vi "Integration Test Launcher.vi"() -> ()   [LabVIEW 2017]
doc: "<License>\nCopyright © 2017 Composed Systems, LLC | All rights reserved\nwww.composed.io\n\nAuthor: Ethan Stern <ethan.stern@composed.io>\n\nThis software is provided \"AS IS\" WITHOUT WARRANTIES, either express or implied, AND IS FOR EDUCATIONAL PURPOSES ONLY.\n</License>"
uses:
  BasicChartBinding/BasicChartBinding.lvclass
  C:/Git/mva-framework/Source/Framework/IViewable/IViewable/IViewable.lvclass
  BasicTerminalBinding/BasicTerminalBinding.lvclass
  MultiSubscriber/MultiSubscriber.lvclass
  ConcreteViewModel/ConcreteViewModel.lvclass
  C:/Git/mva-framework/Source/Framework/IObserver/IObserver/IObserver.lvclass
  C:/Git/mva-framework/Source/Framework/IViewModel/IViewModel/IViewModel.lvclass
  C:/Program Files (x86)/National Instruments/LabVIEW 2017/vi.lib/ActorFramework/Actor/Actor.lvclass
  ValueChangeEventProducer/ValueChangeEventProducer.lvclass
  BasicAutoRegistrationView/BasicAutoRegistrationView.lvclass
  ActorAutoRegistrationView/EventHandlingActor.lvclass
  Source/Framework/IViewModel/IViewModel/IViewModel.lvclass
  C:/Git/mva-framework/Source/Framework/IViewManager/IViewManager/IViewManager.lvclass
  Source/Framework/IViewable/IViewable/View Position Enum.ctl
  Source/Framework/IModel/IModel/IModel.lvclass
  Source/Framework/Mediator/Mediator/Mediator.lvclass
  C:/Git/mva-framework/Source/Framework/IMediator/IMediator/IMediator.lvclass
  <vilib>/ActorFramework/Message Enqueuer/Message Priority.ctl
  ConcreteModel/ConcreteModel.lvclass
  C:/Git/mva-framework/Source/Framework/IModel/IModel/IModel.lvclass
  Source/Framework/Mediator/MediatorBusMonitor/MediatorBusMonitor.lvclass
  C:/Git/mva-framework/Source/Framework/IMediator/IMediatorBusMonitor/IMediatorBusMonitor.lvclass
  TreeActor/TreeActor.lvclass
  MCListboxActor/MCListboxActor.lvclass
  TestApplicationStyle/TestApplicationStyle.lvclass
  <vilib>/Utility/miscctls.llb/LVPointTypeDef.ctl
  gpm_packages/@cs/event-logger/Source/Composed Log/LoggerReference/LoggerReference.lvclass/LoggerReference.ctl
  Source/Framework/IObserver/IObserver/IObserver.lvclass/IObserver.ctl
  Source/Framework/IMediator/IMediator/IMediator.lvclass/IMediator.ctl
  Source/Framework/IViewModel/IViewModel/IViewModel.lvclass/IViewModel.ctl
  Source/Framework/IViewManager/IViewManager Messages/Launch Nested Views Msg/Launch Nested Views Msg.lvclass/Launch Nested Views Msg.ctl
  Source/Framework/IViewManager/IViewManager/IViewManager.lvclass/IViewManager.ctl
  Source/Framework/IViewable/IViewable Messages/Open Front Panel Msg/Open Front Panel Msg.lvclass/Open Front Panel Msg.ctl
  <vilib>/ActorFramework/Message Enqueuer/Message Enqueuer.lvclass/Message Enqueuer.ctl
  Source/Framework/IViewable/IViewable Messages/Set Minimum Panel Size Msg/Set Minimum Panel Size Msg.lvclass/Set Minimum Panel Size Msg.ctl
  52c60252-50fc-4a03-94af-d5c5c5d06c7f.vi
  52c60252-50fc-4a03-94af-d5c5c5d06c7f.vi/977d4e1a-38bf-47f0-b12a-a53eb633355f.vi
  Source/Framework/IObserver/IObserver/Configure Observer Logging.vi
  Source/Framework/IViewModel/IViewModel/Write Startup Model-View Configuration.vi
  Source/Framework/IMediator/IMediator/Configure Mediator.vi
  <vilib>/ActorFramework/Message Enqueuer/Enqueue.vi
  gpm_packages/@cs/event-logger/Source/Composed Log/LoggerReference/Return Aggregate Queues.vi
  gpm_packages/@cs/event-logger/Source/Composed Log/LoggerReference/Add Aggregate Log.vi
  52c60252-50fc-4a03-94af-d5c5c5d06c7f.vi/977d4e1a-38bf-47f0-b12a-a53eb633355f.vi/fc2f1903-e29f-4015-abd4-fc077701cf31.vi
  Source/Framework/IViewManager/IViewManager Messages/Launch Nested Views Msg/Pack Launch Nested Views Msg.vi
  Source/Framework/IViewManager/IViewManager/Write Startup Launch Nested Views Msg.vi
  gpm_packages/@cs/event-logger/Source/Composed Log/LoggerReference/Send Add Sink.vi
  Source/ViewManager/QuadViewManager/QuadViewManager.lvclass
  Source/ViewManager/BoundViewManager/BoundViewManager.lvclass
  Source/ViewManager/TabbedViewManager/TabbedViewManager.lvclass
  Source/Framework/IViewManager/IViewManager/IViewManager.lvclass
  gpm_packages/@cs/event-logger/Source/Text File Sink/Text File Sink.lvclass
  C:/Git/mva-framework/gpm_packages/@cs/event-logger/Source/Composed Log/Log Sink/Log Sink.lvclass
  Source/ViewManager/LeftListboxViewManager/LeftListboxViewManager.lvclass
  Source/Framework/IViewable/IViewable Messages/Open Front Panel Msg/Open Front Panel Msg.lvclass
  C:/Program Files (x86)/National Instruments/LabVIEW 2017/vi.lib/ActorFramework/Message/Message.lvclass
  Source/Framework/IViewable/IViewable Messages/Set Minimum Panel Size Msg/Set Minimum Panel Size Msg.lvclass
  gpm_packages/@cs/event-logger/Source/Composed Log/Application Logger/Launch Worker Loop.vi
  gpm_packages/@cs/event-logger/Source/Composed Log/LoggerReference/Initialize Logger Instance.vi
  <vilib>/ActorFramework/Message Priority Queue/Priority Enqueue.vi
  gpm_packages/@cs/event-logger/Source/Composed Log/LoggerReference/LoggerReference.lvclass
  gpm_packages/@cs/event-logger/Source/Composed Log/IErrorFormat/IErrorFormat.lvclass
  gpm_packages/@cs/event-logger/Source/Composed Log/Log Sink/Log Sink.lvclass
  Source/Framework/IViewable/IApplicationStyle/IApplicationStyle.lvclass
  Source/Framework/IViewManager/IViewManager Messages/Launch Nested Views Msg/Launch Nested Views Msg.lvclass
  <vilib>/ActorFramework/Actor/Actor.lvclass
  Source/Framework/IViewable/IViewable/IViewable.lvclass
  <vilib>/ActorFramework/Message Enqueuer/Message Enqueuer.lvclass
panel:
  out "error out":errorcluster
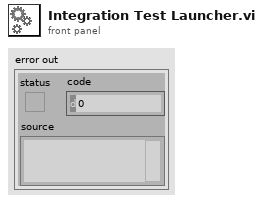
[diagram p1: front panel]
types:
  T1 = typedef "LVPointTypeDef.ctl" = cluster{"Horizontal":i16, "Vertical":i16}
  T2 = typedef "Actor Framework.lvlib/Message Enqueuer.lvclass/Message Priority.ctl" = enum16{"Low", "Normal", "High"}
  T3 = typedef "IViewable.lvlib/IViewable.lvclass/View Position Enum.ctl" = enum16{"Centered", "Maximized", "Minimized", "Custom", "Unchanged"}
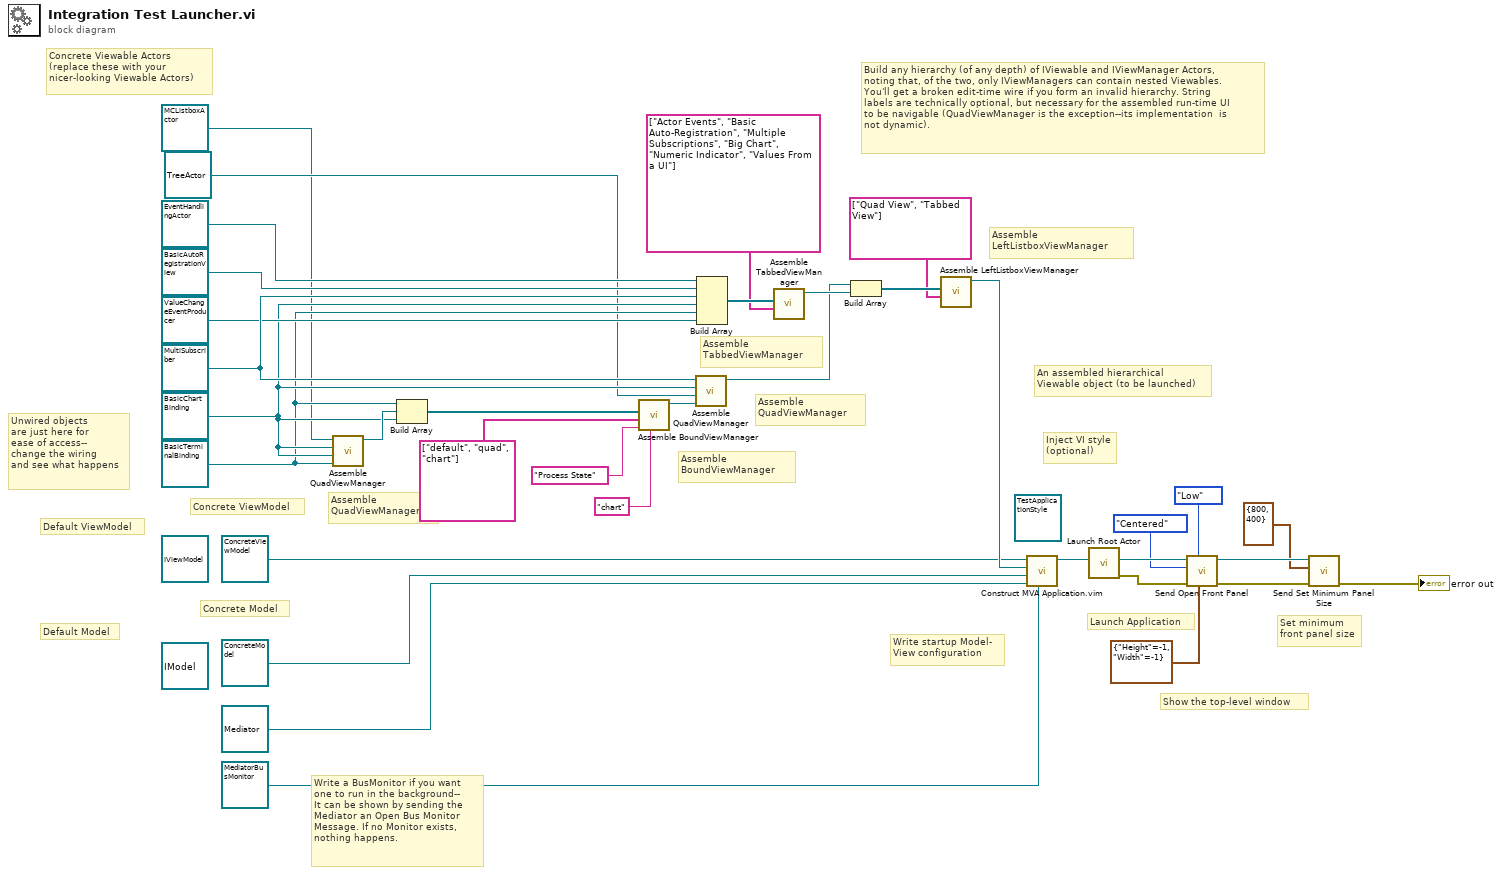
[diagram p0: block diagram]
diagram:
  (unwired) refnum<class "TestApplicationStyle.lvclass"> refnum ("TestApplicationStyle.lvclass")
  (unwired) refnum<class "IModel.lvclass"> refnum ("IModel.lvlib:IModel.lvclass")
  (unwired) refnum<class "IViewModel.lvclass"> refnum ("IController.lvlib:IController.lvclass")
  w28 = refnum<class "MultiSubscriber.lvclass"> refnum ("TestActors.lvlib:ButtonPanel.lvclass")
  w10 = refnum<class "BasicTerminalBinding.lvclass"> refnum ("TestActors.lvlib:NumericCounter.lvclass")
  w12 = refnum<class "BasicChartBinding.lvclass"> refnum ("TestActors.lvlib:RandomDataChart.lvclass")
  # "Set minimum\nfront panel size"
  # "Inject VI style\n(optional)"
  # "An assembled hierarchical\nViewable object (to be launched)"
  # "Assemble\nBoundViewManager"
  # "Assemble\nQuadViewManager"
  # "Assemble\nQuadViewManager"
  # "Assemble\nLeftListboxViewManager"
  # "Assemble\nTabbedViewManager"
  # "Show the top-level window"
  # "Write a BusMonitor if you want\none to run in the background--\nIt can be shown by sending the\nMediator an Open Bus Monitor\nMessage. If no Monitor exists,\nnothing happens."
  # "Unwired objects\nare just here for\nease of access--\nchange the wiring\nand see what happens"
  # "Concrete Model"
  # "Default Model"
  # "Default ViewModel"
  # "Concrete ViewModel"
  # "Concrete Viewable Actors\n(replace these with your\nnicer-looking Viewable Actors)"
  # "Launch Application"
  # "Write startup Model-\nView configuration"
  # "Build any hierarchy (of any depth) of IViewable and IViewManager Actors,\nnoting that, of the two, only IViewManagers can contain nested Viewables.\nYou'll get a broken edit-time wire if you form an invalid hierarchy. String\nlabels are technically optional, but necessary for the assembled run-time UI\nto be navigable (QuadViewManager is the exception--its implementation  is\nnot dynamic)."
  n1 = call "Assemble QuadViewManager.vi"("Bottom-Right View"=w10, "Bottom-Left View"=w12, "Top-Right View"=w12, "Top-Left View"=refnum<class "MCListboxActor.lvclass"> refnum ("TestViewables.lvlib:MCListboxActor.lvclass")) -> ("QuadViewManager out"=w15:refnum<class "QuadViewManager.lvclass">)  [unwired: 7 in]
  n2 = Build Array(w10, w15, w12) -> (w14:refnum<class "IViewable.lvclass">[])
  n3 = call "Assemble BoundViewManager.vi"("Startup View Name (\"\"=None)"="chart" ("Startup View Name (\"\"=None)"), "Selector String Name"="Process State", "Viewable Names"=string[] ["default", "quad", "chart"] ("Insertion Names"), "Bound Viewables"=w14) -> ("BoundViewManager Out"=w16:refnum<class "BoundViewManager.lvclass">)  [unwired: 7 in]
  n4 = call "Assemble QuadViewManager.vi"("Bottom-Right View"=w16, "Bottom-Left View"=refnum<class "TreeActor.lvclass"> refnum ("TestViewables.lvlib:TreeActor.lvclass"), "Top-Right View"=w12, "Top-Left View"=w28) -> ("QuadViewManager out"=w26:refnum<class "QuadViewManager.lvclass">)  [unwired: 7 in]
  n5 = Build Array(refnum<class "EventHandlingActor.lvclass"> refnum ("ActorAutoRegPanel"), refnum<class "BasicAutoRegistrationView.lvclass"> refnum ("AutoRegPanel"), w28, w12, w10, refnum<class "ValueChangeEventProducer.lvclass"> refnum ("TestActors.lvlib:NumericInputs.lvclass")) -> (w34:refnum<class "IViewable.lvclass">[])
  n6 = call "Assemble TabbedViewManager.vi"("View Names"=string[] ["Actor Events", "Basic Auto-Registration", "Multiple Subscriptions", "Big Chart", "Numeric Indicator", "Values From a UI"] ("View Labels"), "Views"=w34) -> ("TabbedViewManager Out"=w31:refnum<class "TabbedViewManager.lvclass">)  [unwired: 9 in]
  n7 = Build Array(w26, w31) -> (w33:refnum<class "IViewManager.lvclass">[])
  n8 = call "Assemble LeftListboxViewManager.vi"("View Names"=string[] ["Quad View", "Tabbed View"] ("View Labels"), "Views"=w33) -> ("LeftListboxViewManager Out"=w32:refnum<class "LeftListboxViewManager.lvclass">)  [unwired: 9 in]
  n9 = call "Construct MVA Application.vim"("MediatorBusMonitor Type"=refnum<class "MediatorBusMonitor.lvclass"> refnum ("Mediator.lvlib:MediatorBusMonitor.lvclass"), "Mediator Type"=refnum<class "Mediator.lvclass"> refnum ("Mediator.lvlib:Mediator.lvclass"), "Model Type"=refnum<class "ConcreteModel.lvclass"> refnum ("TopLevelApplication.lvlib:ConcreteModel.lvclass"), "Startup View Configuration"=w32, "IViewModel In"=refnum<class "ConcreteViewModel.lvclass"> refnum ("TopLevelApplication.lvlib:TopLevelApplication.lvclass")) -> ("IViewModel Out"=w35:refnum<class "ConcreteViewModel.lvclass">)  [unwired: 6 in]
  n10 = call <vilib>:"Launch Root Actor.vi"("Actor"=w35) -> ("error out"=w21:errorcluster, "Actor's Enqueuer"=w23:refnum<class "Message Enqueuer.lvclass">)  [unwired: 9 in]
  n11 = call "Send Open Front Panel.vi"("Custom Window Size"=cluster{"Height":i16, "Width":i16} {"Height"=-1, "Width"=-1} ("Custom Size"), "Message Priority (Normal)"=Message_Priority."Low", "error in (no error)"=w21, "Position"=View_Position_Enum."Centered", "Message Enqueuer"=w23) -> ("error out"=w22:errorcluster, "Message Enqueuer out"=w4:refnum<class "Message Enqueuer.lvclass">)  [unwired: 5 in]
  n12 = call "Send Set Minimum Panel Size.vi"("error in (no error)"=w22, "Minimum Size"=T1 {"Horizontal"=800, "Vertical"=400}, "Message Enqueuer"=w4) -> ("error out"=→"error out":errorcluster)  [unwired: 7 in, 1 out]
